vi "connect_objects.vi"(8 "to object terminal index":i32, 9 "to object id":string, 10 "from object terminal index":i32, 11 "from object id":string) -> (0 "error out":errorcluster)   [LabVIEW 2026]
doc: "Connects two terminals of two objects with a wire on the block diagram of a labview vi. To get a new VI use \"new vi\" to add objects to a vi use \"add object\". If a frontpanel control/indicator reference is passed to this function, it will automatically use the corresponding terminal on the block diagram for wiring. Use get_object_terminals before wiring to find out which terminals to wire."
uses:
  G-AI Core/G-AI Core.lvlib
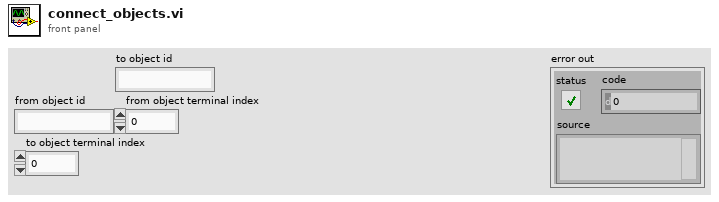
[diagram p1: front panel]
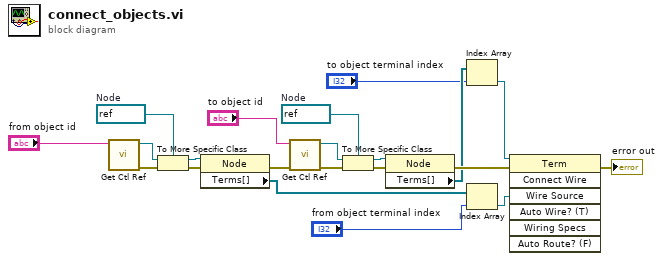
[diagram p0: block diagram]
diagram:
  w14 = refnum<vi> refnum  # Node
  w19 = refnum<vi> refnum  # Node
  n1 = call "Get Ctl Ref.vi"("ctl id"="from object id") -> ("error out"=w18:errorcluster, "ctl ref"=w21:refnum<vi>)  [unwired: 9 in]
  n2 = To More Specific Class(target class=w19, reference=w21, error in=w18) -> (specific class reference=w20:refnum<vi>, error out=w17:errorcluster)
  n3 = property class="Node"(reference=w20, error in=w17) -> (error out=w11:errorcluster, "Terms[]"=w9:refnum<vi>[])  [unwired: 1 out]
  n4 = call "Get Ctl Ref.vi"("error in"=w11, "ctl id"="to object id") -> ("error out"=w15:errorcluster, "ctl ref"=w12:refnum<vi>)  [unwired: 8 in]
  n5 = To More Specific Class(target class=w14, reference=w12, error in=w15) -> (specific class reference=w13:refnum<vi>, error out=w16:errorcluster)
  n6 = property class="Node"(reference=w13, error in=w16) -> (error out=w10:errorcluster, "Terms[]"=w8:refnum<vi>[])  [unwired: 1 out]
  n7 = Index Array(array=w8, index="to object terminal index") -> (element=w3:refnum<vi>)
  n8 = Index Array(array=w9, index="from object terminal index") -> (element=w2:refnum<vi>)
  n9 = invoke class="Term" method="Connect Wire"(reference=w3, error in=w10, "Wire Source"=w2) -> (error out=→"error out":errorcluster)  [unwired: 4 in, 6 out]
